vi "Key - Adjust Names For Report.vi"(11 "Parameters":string[][](array[string])=[["Sequence Number", "1", "2", "", "", "", "", "", "", "", "", "", "", "", "", "", ""], ["Ramp Rate", "200", "100", "", "", "", "", "", "", "", "", "", "", "", "", "", ""], ["Target Temperature", "70", "50", "", "", "", "", "", "", "", "", "", "", "", "", "", ""], ["Hold Time", "00:25", "00:00", "", "", "", "", "", "", "", "", "", "", "", "", "", ""], ["Additional WPS", "AddWPS106", "AddWPS107", "", "", "", "", "", "", "", "", "", "", "", "", "", ""], ["Rev.", "1", "2", "", "", "", "", "", "", "", "", "", "", "", "", "", ""], ["Name", "Temperature Controller", "Temperature Module (NI)", "Temperature Module (NI)", "", "", "", "", "", "", "", "", "", "", "", "", ""], ["Model", "ET-3504", "NI-9211", "NI-9211", "", "", "", "", "", "", "", "", "", "", "", "", ""], ["Serial No.", "E123-01", "12F0001", "12F0002", "", "", "", "", "", "", "", "", "", "", "", "", ""], ["Last Cal. Date", "23-11-2013", "01-01-2014", "02-02-2014", "", "", "", "", "", "", "", "", "", "", "", "", ""], ["Next Cal. Due Date", "22-12-2015", "30-12-2015", "28-02-2015", "", "", "", "", "", "", "", "", "", "", "", "", ""], ["Equipment ID", "ET-3504 01", "NI-9211 01", "NI-9211 02", "", "", "", "", "", "", "", "", "", "", "", "", ""], ["Notice Period", "30", "30", "60", "", "", "", "", "", "", "", "", "", "", "", "", ""], ["Cal. Required", "-1", "-1", "-1", "", "", "", "", "", "", "", "", "", "", "", "", ""], ["WPS/Ref", "WPS104105", "", "", "", "", "", "", "", "", "", "", "", "", "", "", ""], ["Rev", "", "", "", "", "", "", "", "", "", "", "", "", "", "", "", ""], ["Hold Temperature", "70", "", "", "", "", "", "", "", "", "", "", "", "", "", "", ""], ["WPS Details Temperature Units", "°C", "", "", "", "", "", "", "", "", "", "", "", "", "", "", ""], ["Hold Time (HH:MM)", "00:25", "", "", "", "", "", "", "", "", "", "", "", "", "", "", ""], ["Inactive", "F", "", "", "", "", "", "", "", "", "", "", "", "", "", "", ""], ["Furnace Serial No", "A1234A1", "", "", "", "", "", "", "", "", "", "", "", "", "", "", ""], ["Last Calibration Date", "23-11-2013", "", "", "", "", "", "", "", "", "", "", "", "", "", "", ""], ["Next Calibration Due Date", "22-12-2015", "", "", "", "", "", "", "", "", "", "", "", "", "", "", ""], ["Channel to Probe Mapping", "1", "2", "3", "4", "5", "6", "7", "8", "9", "10", "11", "12", "13", "14", "15", "16"], ["Start Holding Time & Date", "2015-02-09 10:37:44", "", "", "", "", "", "", "", "", "", "", "", "", "", "", ""], ["End Holding Time & Date", "2015-02-09 11:02:44", "", "", "", "", "", "", "", "", "", "", "", "", "", "", ""], ["Recorded Hold Time (hh:mm)", "0:25", "", "", "", "", "", "", "", "", "", "", "", "", "", "", ""], ["Start Holding Temperature °C", "70", "", "", "", "", "", "", "", "", "", "", "", "", "", "", ""], ["End Holding Temperature °C", "70", "", "", "", "", "", "", "", "", "", "", "", "", "", "", ""], ["Difference in Holding Temperature °C", "0.0", "", "", "", "", "", "", "", "", "", "", "", "", "", "", ""], ["Permitted Holding Temperature Difference °C", "8", "", "", "", "", "", "", "", "", "", "", "", "", "", "", ""], ["Permitted Holding Time (min)", "30", "", "", "", "", "", "", "", "", "", "", "", "", "", "", ""], ["Process Status", "Fail", "", "", "", "", "", "", "", "", "", "", "", "", "", "", ""]]) -> (3 "output array":string[][](array[string]))   [LabVIEW 2013]
panel:
  in  "Replace":string[](array[string])=["Hold Time Duration", "Equipment Serial No.", "Last Calibration Date", "Next Calibration Date", "Calibration Required", "WPS Rev", "Additional WPS Number", "Last Inspection Date", "Next Inspection Due Date", "Permitted Temp Diff", "Permitted Time Diff"]
  in  "Search":string[](array[string])=["Hold Time", "Serial No.", "Last Cal. Date", "Next Cal. Due Date", "Cal. Required", "Rev", "Additional WPS", "Last Calibration Date", "Next Calibration Due Date", "Permitted Holding Temperature Difference °C", "Permitted Holding Time (min)"]
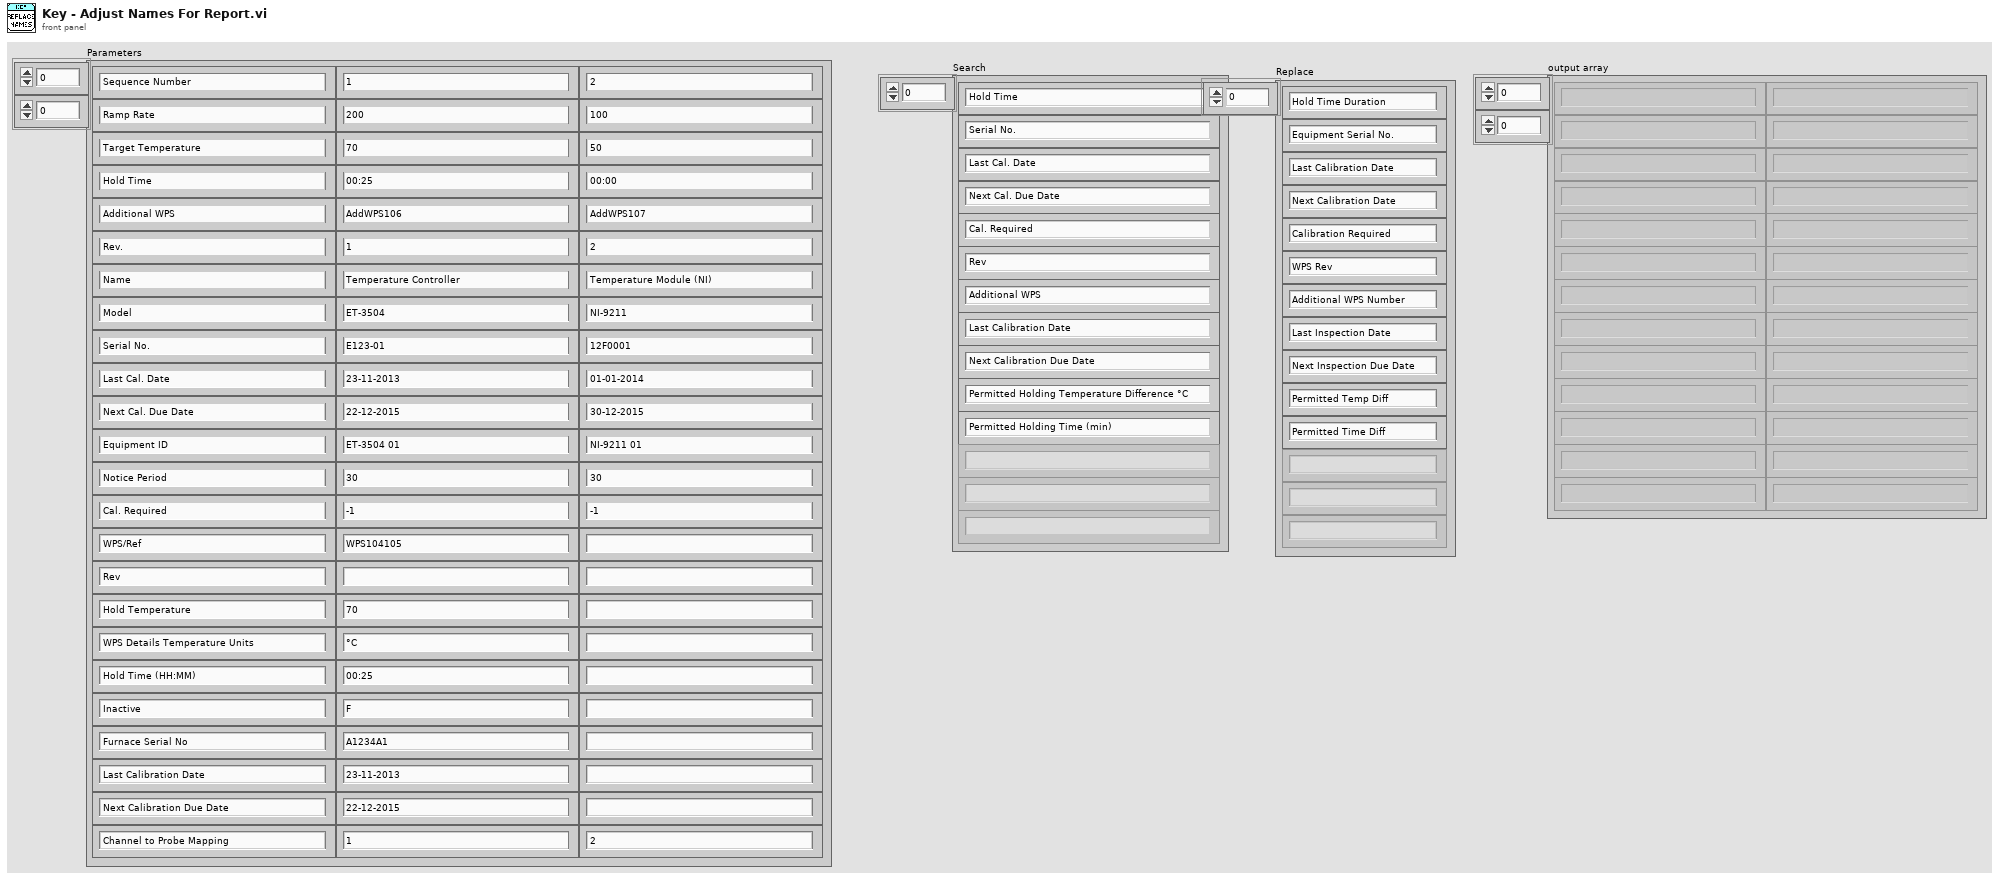
[diagram p1: front panel]
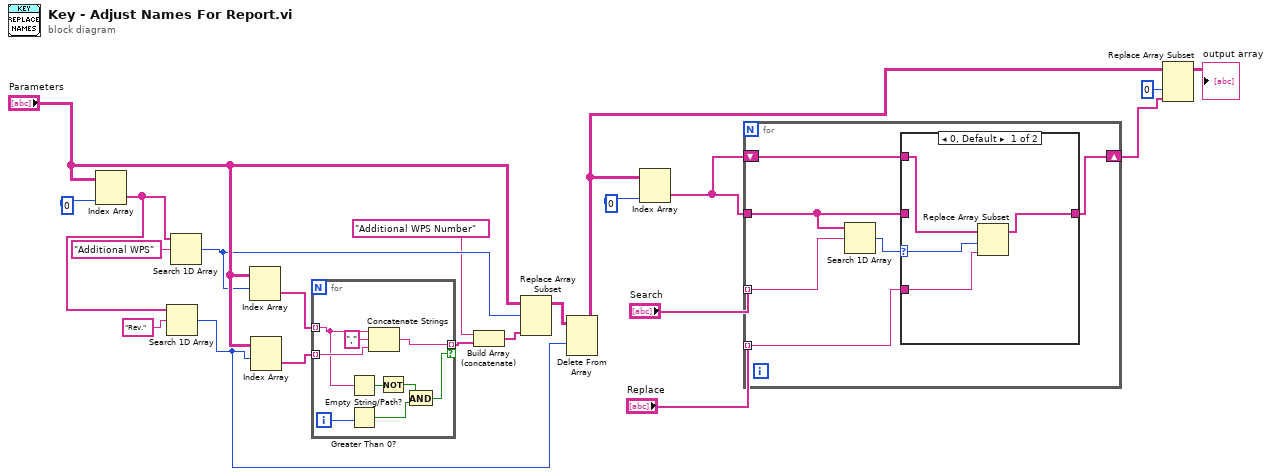
[diagram p0: block diagram]
diagram:
  n1 = Index Array(array="Parameters", index (col)=0 ("disabled index (col)")) -> (element=w12:string[])  [unwired: 1 in]
  n2 = Search 1D Array(1D array=w12, element="Rev.") -> (index of element=w2:i32)  [unwired: 1 in]
  n3 = Search 1D Array(1D array=w12, element="Additional WPS") -> (index of element=w7:i32)  [unwired: 1 in]
  n4 = Index Array(array="Parameters", index (row)=w7) -> (element=w10:string[])  [unwired: 1 in]
  n5 = Index Array(array="Parameters", index (row)=w2) -> (element=w9:string[])  [unwired: 1 in]
  n6 = for {
    tunnel: w10 -> [w26] mode=indexing
    tunnel: w9 -> [w29] mode=indexing
    tunnel: [w28] -> w6 mode=indexing if=w22
    i -> [w27]
    n7 = Empty String/Path?(string/path=w26) -> (empty?=w25:bool)
    n8 = Greater Than 0?(x=w27) -> (x > 0?=w23:bool)
    n9 = Concatenate Strings(w26, "," ("string"), w29) -> (w28:string)
    n10 = Not(x=w25) -> (.not. x?=w24:bool)
    n11 = And(x=w24, y=w23) -> (x .and. y?=w22:bool)
  }
  n12 = Build Array (concatenate)("Additional WPS Number", w6) -> (w4:string[])
  n13 = Replace Array Subset(array="Parameters", new element=w4, index (row)=w7) -> (w3:string[][])  [unwired: 1 in]
  n14 = Delete From Array(array=w3, index (row)=w2) -> (array with subset deleted=w1:string[][])  [unwired: 2 in, 1 out]
  n15 = Index Array(array=w1, index (col)=0 ("disabled index (col)")) -> (element=w15:string[])  [unwired: 1 in]
  n16 = for {
    tunnel: "Search" -> [w36] mode=indexing
    tunnel: "Replace" -> [w34] mode=indexing
    shift-right: [w33] -> w16
    shift-left: w15 -> [w31]
    tunnel: w15 -> [w32]
    n17 = Search 1D Array(1D array=w32, element=w36) -> (index of element=w35:i32)  [unwired: 1 in]
    n18 = case shown="0, Default" w35 {
      selector: w35 -> [w40 _]
      tunnel: w32 -> [_ _]
      tunnel: w34 -> [w39 _]
      tunnel: [w38 w41] -> w33
      tunnel: w31 -> [w37 w41]
      frame 0, Default {
        n19 = Replace Array Subset(array=w37, new element=w39, index=w40) -> (w38:string[])
      }
      frame -1 {
      }
    }
  }
  n20 = Replace Array Subset(array=w1, new element=w16, index (col)=0 ("disabled index (col)")) -> (→"output array":string[][])  [unwired: 1 in]
